vi "Build_tdms_group_name.vi"(9 "SiPM Y":i32, 10 "SiPM X":i32) -> (3 "Group_name":string)   [LabVIEW 2019]
uses:
  SiPM_Tests_Global_Var.vi
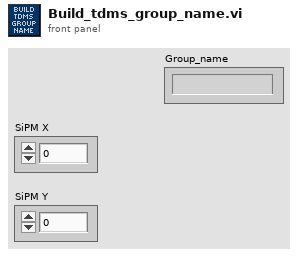
[diagram p1: front panel]
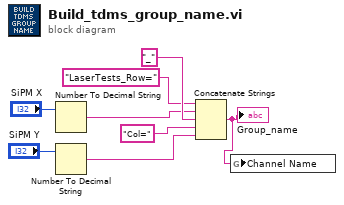
[diagram p0: block diagram]
diagram:
  n1 = Number To Decimal String(number="SiPM X") -> (decimal integer string=w5:string)  [unwired: 1 in]
  n2 = Number To Decimal String(number="SiPM Y") -> (decimal integer string=w8:string)  [unwired: 1 in]
  n3 = Concatenate Strings("LaserTests_Row=" ("group name in (Untitled)"), w5, "_" ("string"), "Col=" ("group name in (Untitled)"), w8) -> (w1:string)
  "Group_name" <- w1
  n4 = global write "SiPM_Tests_Global_Var.vi" "Channel Name"(w1) -> ()
